vi "Format Output CSV.vi"(10 "logData":T1, 11 "String":string) -> (3 "Array":string[](array[string]))   [LabVIEW 2012]
uses:
  Nufi/Newfi LDN/subVI/logData.ctl
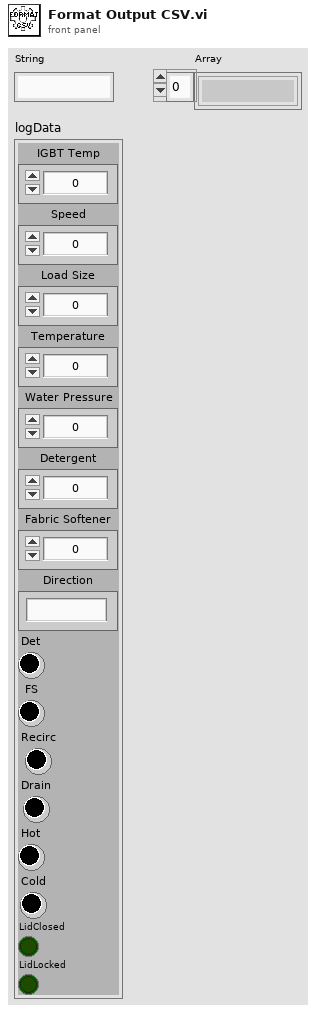
[diagram p1: front panel]
types:
  T1 = typedef "logData.ctl" = cluster{"IGBT Temp":u8, "Speed":u32, "Load Size":u32, "Temperature":u8, "Water Pressure":u32, "Detergent":u32, "Fabric Softener":u32, "Direction":string, "Det":bool, "FS":bool, "Recirc":bool, "Drain":bool, "Hot":bool, "Cold":bool, "LidClosed":bool, "LidLocked":bool}
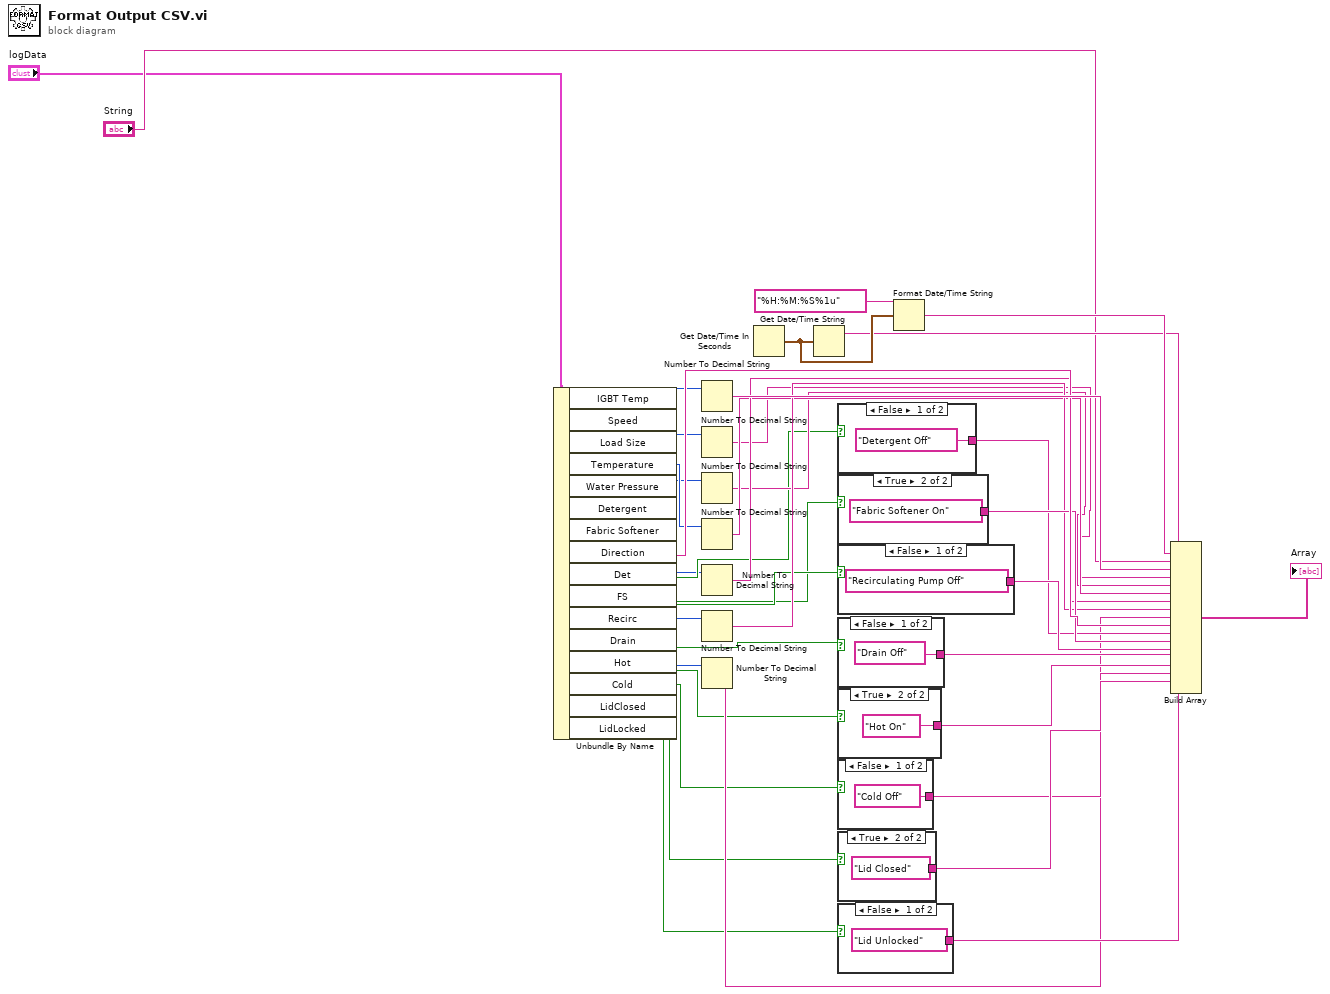
[diagram p0: block diagram]
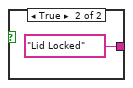
[diagram p2: hidden frame]
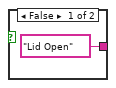
[diagram p3: hidden frame]
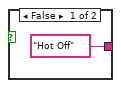
[diagram p4: hidden frame]
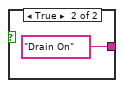
[diagram p5: hidden frame]
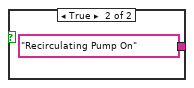
[diagram p6: hidden frame]
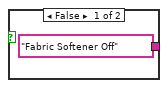
[diagram p7: hidden frame]
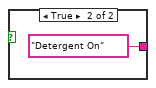
[diagram p8: hidden frame]
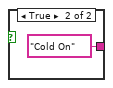
[diagram p9: hidden frame]
diagram:
  n1 = Unbundle By Name("logData") -> ("IGBT Temp"=w2:u8, "Speed"=w3:u32, "Load Size"=w4:u32, "Temperature"=w5:u8, "Water Pressure"=w6:u32, "Detergent"=w7:u32, "Fabric Softener"=w8:u32, "Direction"=w34:string, "Det"=w9:bool, "FS"=w10:bool, "Recirc"=w11:bool, "Drain"=w12:bool, "Hot"=w13:bool, "Cold"=w14:bool, "LidClosed"=w15:bool, "LidLocked"=w16:bool)
  n2 = Number To Decimal String(number=w2) -> (decimal integer string=w35:string)  [unwired: 1 in]
  n3 = Number To Decimal String(number=w3) -> (decimal integer string=w17:string)  [unwired: 1 in]
  n4 = Number To Decimal String(number=w4) -> (decimal integer string=w18:string)  [unwired: 1 in]
  n5 = Number To Decimal String(number=w5) -> (decimal integer string=w19:string)  [unwired: 1 in]
  n6 = Number To Decimal String(number=w6) -> (decimal integer string=w20:string)  [unwired: 1 in]
  n7 = Number To Decimal String(number=w7) -> (decimal integer string=w21:string)  [unwired: 1 in]
  n8 = Number To Decimal String(number=w8) -> (decimal integer string=w22:string)  [unwired: 1 in]
  n9 = Get Date/Time In Seconds() -> (seconds since 1Jan1904=w36:timestamp)
  n10 = Get Date/Time String(seconds (now)=w36) -> (date string=w32:string)  [unwired: 2 in, 1 out]
  n11 = case shown="False" w9 {
    tunnel: ["Detergent Off" "Detergent On"] -> w23
    frame False {
    }
    frame True {
    }
  }
  n12 = case shown="True" w10 {
    tunnel: ["Fabric Softener Off" "Fabric Softener On"] -> w24
    frame False {
    }
    frame True {
    }
  }
  n13 = case shown="False" w11 {
    tunnel: ["Recirculating Pump Off" "Recirculating Pump On"] -> w25
    frame False {
    }
    frame True {
    }
  }
  n14 = case shown="False" w12 {
    tunnel: ["Drain Off" "Drain On"] -> w26
    frame False {
    }
    frame True {
    }
  }
  n15 = case shown="True" w13 {
    tunnel: ["Hot Off" "Hot On"] -> w27
    frame False {
    }
    frame True {
    }
  }
  n16 = case shown="False" w14 {
    tunnel: ["Cold Off" "Cold On"] -> w28
    frame False {
    }
    frame True {
    }
  }
  n17 = case shown="True" w15 {
    tunnel: ["Lid Open" "Lid Closed"] -> w29
    frame False {
    }
    frame True {
    }
  }
  n18 = case shown="False" w16 {
    tunnel: ["Lid Unlocked" "Lid Locked"] -> w30
    frame False {
    }
    frame True {
    }
  }
  n19 = Format Date/Time String(time format string (%c)="%H:%M:%S%1u", seconds (now)=w36) -> (date/time string=w38:string)  [unwired: 1 in]
  n20 = Build Array(w32, w38, "String", w35, w17, w18, w19, w20, w21, w22, w34, w23, w24, w25, w26, w27, w28, w29, w30) -> (→"Array":string[])
